vi "Wait For Acquisition Complete.vi"(8 "error in (no error)":errorcluster, 10 "Maximum Time (10000 ms)":i32=10000, 11 "VISA resource name":refnum<visa-resource-name>) -> (0 "error out":errorcluster, 3 "VISA resource name out":refnum<visa-resource-name>)   [LabVIEW 2017, in "Keysight B2980 Series.lvlib"]
doc: "Waits for the acquisition to finish. This VI should be called after Initiate VI and before Fetch Measurement VI.\n\n<B>Note:</B> \nUse this VI only with other low-level VIs. The high-level VIs automatically incorporate this functionality. This VI does not check the instrument status."
uses:
  Keysight B2980 Series.lvlib
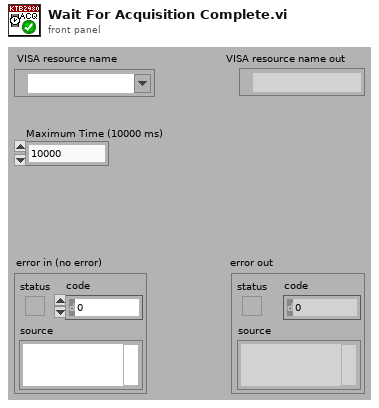
[diagram p1: front panel]
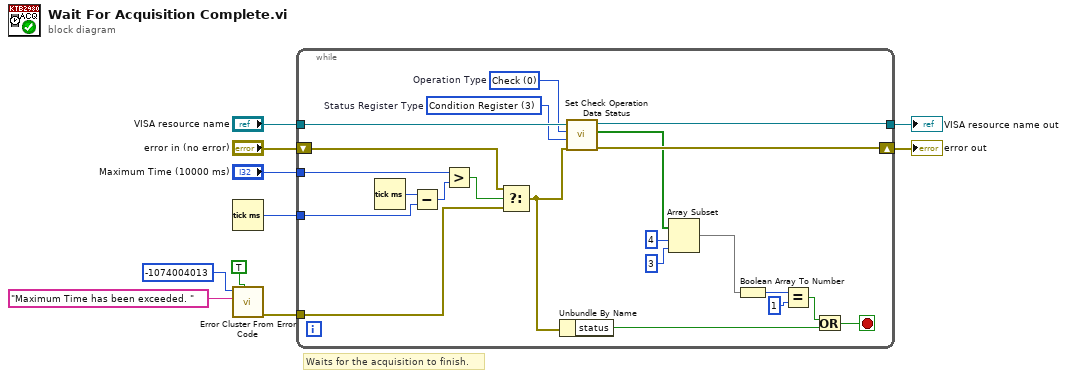
[diagram p0: block diagram]
diagram:
  # "Waits for the acquisition to finish."
  n1 = Tick Count (ms)() -> (millisecond timer value=w6:u32)
  n2 = call <vilib>:"Error Cluster From Error Code.vi"("show call chain? (False)"=TRUE, "error message (\"\")"="Maximum Time has been exceeded. " ("error message (\"\")"), "error code (0)"=-1074004013) -> ("error out"=w8:errorcluster)  [unwired: 1 in, 5 out]
  n3 = while {
    tunnel: w8 -> [w24]
    tunnel: w6 -> [w28]
    tunnel: "Maximum Time (10000 ms)" -> [w27]
    tunnel: "VISA resource name" -> [w16]
    shift-right: [w18] -> w1
    shift-left: "error in (no error)" -> [w25]
    tunnel: [w19] -> w2
    stop <- w23 stop-if-true
    w13 = 0 items=["Check", "Set"]  # Operation Type
    w14 = 3 items=["Enable Register", "Negative Transition Filter Register", "Positive Transition Filter Register", "Condition Register", "Event Register"]  # Status Register Type
    n4 = Tick Count (ms)() -> (millisecond timer value=w29:u32)
    n5 = Subtract(x=w29, y=w28) -> (x-y=w26:u32)
    n6 = Greater?(x=w27, y=w26) -> (0:w21:bool)
    n7 = Select(t=w25, s=w21, f=w24) -> (s? t:f=w15:errorcluster)
    n8 = Unbundle By Name(w15) -> ("status"=w20:bool)
    n9 = call "Set Check Operation Data Status.vi"("error in (no error)"=w15, "Status Register Type (0: Enable Register)"=w14, "Operation Type (0: Check)"=w13, "VISA resource name"=w16) -> ("error out"=w18:errorcluster, "Register Status"=w17:bool[], "VISA resource name out"=w19:refnum<visa-resource-name>)  [unwired: 1 in, 4 out]
    n10 = Array Subset(array=w17, index=4, length=3) -> (w32:bool[])
    n11 = Boolean Array To Number(Boolean array=w32) -> (number=w31:u32)
    n12 = Equal?(x=w31, y=u32 1) -> (x = y?=w22:bool)
    n13 = Or(x=w22, y=w20) -> (x .or. y?=w23:bool)
  }
  "VISA resource name out" <- w2
  "error out" <- w1
